vi "Write FIFO (Two Channels).vi"(0 "data in":u32[](array[numeric]), 1 "fifo 0":refnum<k21>, 2 "fifo 1":refnum<k21>, 5 "enable":bool[](array[boolean]), 9 "input valid":bool, 12 "fifo 0 enable":bool, 13 "fifo 1 enable":bool) -> (14 "ready for input":bool)   [LabVIEW 2020]
doc: "Writes data to two 32-bit FIFOs. This VI is a wrapper around the LabVIEW FPGA FIFO Write method. This VI exposes handshaking signals that inform the user when the FIFOs are ready to accept new data.\n\n<B>Input Parameters</B>\n\n<B>data in</B> is the data to be written to the FIFO.\n\n<B>enabled</B> specifies which streams are enabled.\n\n<B>input valid</B> specifies when 'data in' is valid.\n\n<B>reset</B> the LabVIEW FPGA FIFO.\n\n<B>fifo 0</B> is the reference to the FIFO to which data received on channel 0 will be written to.\n\n<B>fifo 1</B> is the reference to the FIFO to which data received on channel 1 will be written to.\n\n<B>Output Parameters</B>\n\n<B>ready for input</B> is a flow control signal that indicates whether the Write FIFO VI is ready to accept new data."
uses:
  <vilib>/rvi/DataTransferAndStorage/Container/Common/niFpgaContainerExecOnDevCompGetState.vi
  <vilib>/rvi/Emulation/niFpgaEmulationIsFPGAContextNoSignature.vi
  <vilib>/rvi/Emulation/niFpgaSctlEmulationGetInTimedLoop.vi
  <vilib>/rvi/errors/niFpgaSetErrorForExecOnDevCompSimple.vi
  <vilib>/rvi/eio/common/nirviEmuReportErrorAndStop.vi
  <vilib>/rvi/DataTransferAndStorage/Container/Common/niFpgaContainerGetUniqueNameForEmu.vi
  <vilib>/rvi/FIFO/Fifo_Resource/nirvififoEmulationSetSize.vi
  <vilib>/rvi/FIFO/Fifo_Resource/nirviFifoEmulationQueueMgr.vi
  <instcachedir>/0/nirviFifoEmulationQueueMgr_E5CAEC123FF24DC58D834DCA3CDAA9B5.lvgen/nirviFifoEmulationQueueMgr_E5CAEC123FF24DC58D834DCA3CDAA9B5_004.vi
  <vilib>/rvi/FIFO/Fifo_Resource/nirvififoEmulationDetermineInputValidOut.vi
  <vilib>/rvi/FIFO/Fifo_Resource/nirvififoEmulationCreateLock.vi
  <vilib>/rvi/Emulation/niFpgaProcessEmulError.vi
  <vilib>/rvi/FIFO/Fifo_Resource/nirvififoEmulationObtainLock.vi
  <vilib>/rvi/FIFO/Fifo_Resource/nirvififoEmulationReleaseLock.vi
  <vilib>/rvi/occurrence/nirviWaitOnOccurrenceBase.vi
  <vilib>/rvi/errors/nirviReportUnexpectedCaseInternalError.vi
  <vilib>/rvi/errors/nirviReportUnexpectedCaseInternalError (U32).vi
  <vilib>/Utility/error.llb/Clear Errors.vi
  <vilib>/rvi/interface/RandomDataEmulation/niFpgaRandomDataHandleErrors.vi
  <vilib>/rvi/DataTransferAndStorage/Container/XNode/niFpgaContainer.xnode
  <vilib>/rvi/FIFO/Fifo_Resource/niFpgaFifoEmulationRefIn.vi
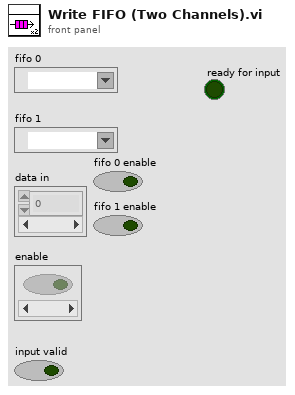
[diagram p1: front panel]
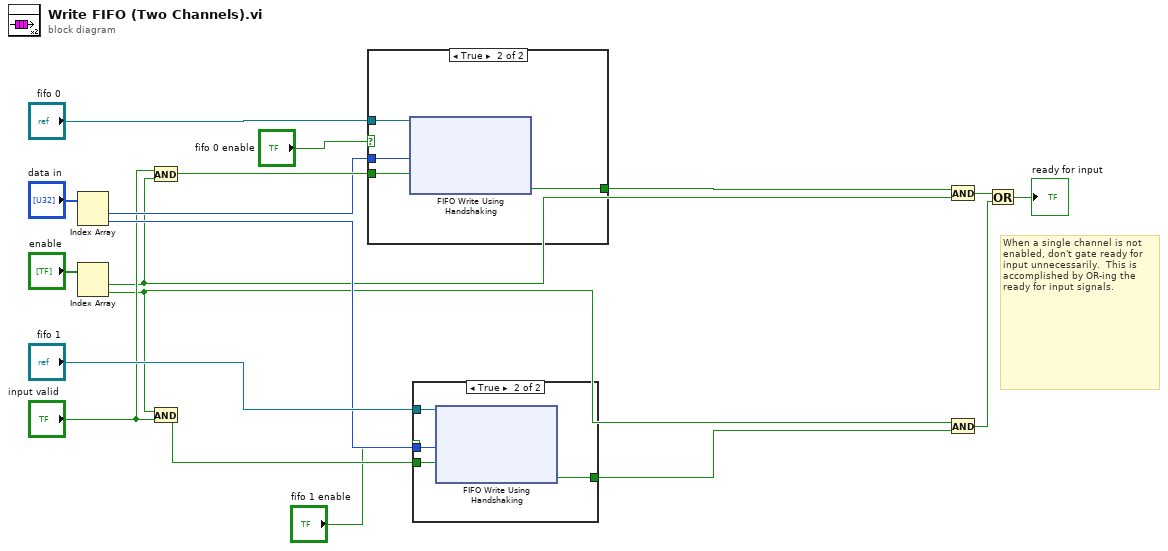
[diagram p0: block diagram]
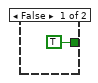
[diagram p2: hidden frame]
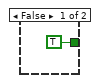
[diagram p3: hidden frame]
diagram:
  # "When a single channel is not enabled, don't gate ready for input unnecessarily.  This is accomplished by OR-ing the ready for input signals."
  n1 = Index Array(array="data in") -> (element #1=w12:u32, element #2=w10:u32)  [unwired: 2 in]
  n2 = Index Array(array="enable") -> (element #1=w8:bool, element #2=w3:bool)  [unwired: 2 in]
  n3 = And(x="input valid", y=w8) -> (x .and. y?=w14:bool)
  n4 = And(x=w3, y="input valid") -> (x .and. y?=w11:bool)
  n5 = case shown="True" "fifo 0 enable" {
    tunnel: "fifo 0" -> [_ w23]
    tunnel: w14 -> [_ w22]
    tunnel: [TRUE ("Ready for Input") w21] -> w13
    tunnel: w12 -> [_ w20]
    frame False {
    }
    frame True {
      n6 = xnode "FIFO Write Using Handshaking"("Element"=w20, "Input Valid"=w22, "FIFO In"=w23) -> ("Ready for Input"=w21:bool)  [unwired: 1 out]
    }
  }
  n7 = case shown="True" "fifo 1 enable" {
    tunnel: "fifo 1" -> [_ w28]
    tunnel: w11 -> [_ w27]
    tunnel: w10 -> [_ w26]
    tunnel: [TRUE ("Ready for Input") w25] -> w4
    frame False {
    }
    frame True {
      n8 = xnode "FIFO Write Using Handshaking"("Element"=w26, "Input Valid"=w27, "FIFO In"=w28) -> ("Ready for Input"=w25:bool)  [unwired: 1 out]
    }
  }
  n9 = And(x=w13, y=w8) -> (x .and. y?=w7:bool)
  n10 = And(x=w3, y=w4) -> (x .and. y?=w6:bool)
  n11 = Or(x=w7, y=w6) -> (x .or. y?=→"ready for input":bool)
